vi "Initialize.vi"(0 "Cal Standard Base in":refnum<class "Cal Standard Base.lvclass">, 11 "error in (no error)":errorcluster) -> (4 "Cal Standard Base out":refnum<class "Cal Standard Base.lvclass">, 6 "Found":bool, 15 "error out":errorcluster)   [LabVIEW 2023, in "RFFixtureCharact.Instruments.lvlib" / "Cal Standard Base.lvclass"]
uses:
  Cal Standard Base.lvclass
  Type Definitions/One-Port Cal Standard.ctl
  Type Definitions/One-Port Charact Data.ctl
  Type Definitions/Standard Type.ctl
  Cal Standard Base.lvclass/Cal Standard Base.ctl
  Properties/Write Instrument Info.vi
  Properties/Write Path Connection Map.vi
  Properties/Write One-Port Cal Standards.vi
  RFFixtureCharact.Instruments.lvlib
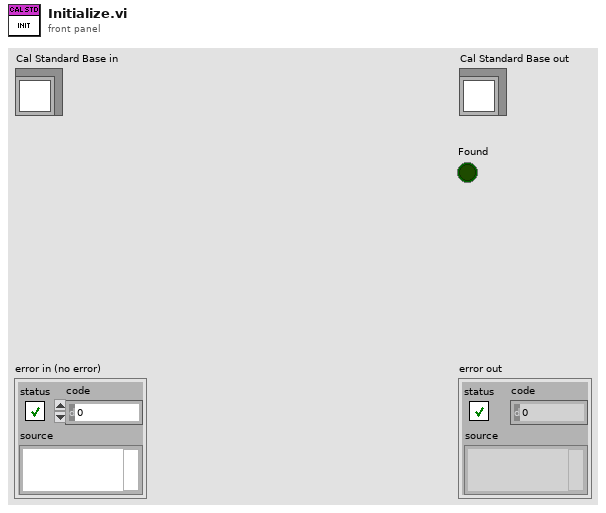
[diagram p1: front panel]
types:
  T1 = typedef "RFFixtureCharact.Instruments.lvlib/One-Port Cal Standard.ctl" = cluster{"Port Name":string, "Charact Data":T2[]}
  T2 = typedef "RFFixtureCharact.Instruments.lvlib/One-Port Charact Data.ctl" = cluster{"Standard Type":T3, "Frequencies":dbl[], "S11":cdb[]}
  T3 = typedef "RFFixtureCharact.Instruments.lvlib/Standard Type.ctl" = enum16{"Short", "Open", "Load"}
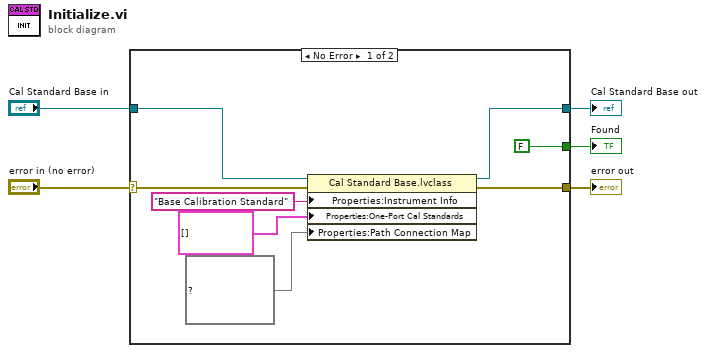
[diagram p0: block diagram]
diagram:
  n1 = case shown="No Error" "error in (no error)" {
    selector: "error in (no error)" -> [w12 w15]
    tunnel: [w10 w15] -> w4
    tunnel: [w9 w14] -> w2
    tunnel: "Cal Standard Base in" -> [w11 w14]
    tunnel: [FALSE ("Found") _] -> w1
    frame No Error {
      n2 = property class="Cal Standard Base.lvclass"(reference=w11, error in=w12, "Properties:Instrument Info"="Base Calibration Standard", "Properties:One-Port Cal Standards"=T1[] [] ("One-Port Cal Standards"), "Properties:Path Connection Map"=map{string, string[]} {} ("Path Connection Map")) -> (reference out=w9:refnum<class "Cal Standard Base.lvclass">, error out=w10:errorcluster)
    }
    frame Error {
    }
  }
  "error out" <- w4
  "Cal Standard Base out" <- w2
  "Found" <- w1
